vi "AG33XXX.constructor.vi"(0 "name":string, 2 "data in":string, 5 "error in (no error)":errorcluster) -> (14 "i ref out":refnum<vi>, 16 "data out":string, 19 "error out":errorcluster)   [LabVIEW 2014, in "AG33XXX.lvlib"]
doc: "Constructor of the AG33XXX class.\n\nLicense Agreement for this software:\n\nCopyright (C)\nGesellschaft für Schwerionenforschung, GSI\nPlanckstr. 1\n64291 Darmstadt\nGermany\n\nContact: D.Beck@gsi.de \n\nThis program is free software; you can redistribute it and/or modify it under the terms of the \nGNU General Public License as published by the Free Software Foundation; either version 2 of \nthe license, or (at your option) any later version.\n\nThis program is distributed in the hope that it will be useful, but WITHOUT ANY WARRANTY; \nwithout even the implied warranty of MERCHANTABILITY or FITNESS FOR A PARTICULAR PURPOSE. See the GNU General License for more details (http://www.gnu.org).\n\nGesellschaft für Schwerionenforschung, GSI\nPlanckstr. 1, 64291 Darmstadt, Germany\nFor all questions and ideas contact: M.Richter@gsi.de, H.Brand@gsi.de or D.Beck@gsi.de.\nLast update: 16-JUN-2004"
uses:
  AG33XXX.lvlib
  CS_Core/CSApplicationBaseClasses/DeviceBase/DeviceBase.myEventNames.ctl
  CS_Core/CSApplicationBaseClasses/AFGBase/AFGBase.myEventNames.ctl
  CS_Core/CSSystem/CSSystemLib/CSSystemLib.lvlib
  CS_Core/CSApplicationBaseClasses/AFGBase/AFGBase.lvlib
  CS_Core/CSApplicationBaseClasses/DeviceBase/DeviceBase.lvlib
  CS_Core/BaseProcess/BaseProcess.lvlib
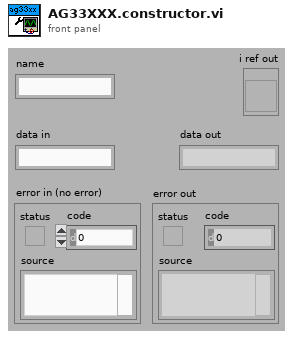
[diagram p1: front panel]
types:
  T1 = enum16{"SetAttribute", "GetAttribute", "CreateAttribute", "DestroyAttribute", "DestroyAllAtributes"}
  T2 = typedef "AFGBase.lvlib/AFGBase.myEventNames.ctl" = enum16{"lvmsg://SetFrequency", "lvmsg://GetFrequency", "lvmsg://SetAmplitude", "lvmsg://GetAmplitude", "lvmsg://SetPhase", "lvmsg://GetPhase", "lvmsg://SetDCOffset", "lvmsg://GetDCOffset", "lvmsg://SetWaveformType", "lvmsg://GetWaveformType", "lvmsg://SetOutputEnabled", "lvmsg://GetOutputEnabled", "lvmsg://SetWaveform", "lvmsg://GetWaveform", "lvmsg://SetTrigger", "lvmsg://GetTrigger", "lvmsg://SetWaveformParams", "lvmsg://GetWaveformParams"}
  T3 = typedef "DeviceBase.lvlib/DeviceBase.myEventNames.ctl" = enum16{"lvmsg://Initialize", "lvmsg://Close", "lvmsg://Configure", "lvmsg://Reset", "lvmsg://IDQuery"}
  T4 = typedef "BaseProcess.lvlib/BaseProcess.i attribute.ctl" = cluster{"EventStatus":string, "EventError":i32, "PresetEvtWatchD":i32, "PresetPdcWatchD":i32, "EventTimeout":i32, "PeriodicInterval":i32, "Interface":string[], "Address":string[], "Special":string[], "PeriodicError":i32, "PeriodicStatus":string, "SuperProc":string, "Descriptors":T5[], "CaseRef":refnum<vi>, "PdcRef":refnum<vi>, "Thread Ref":refnum<vi>, "eventErrorID":i32, "eventStatusID":i32, "periodicErrorID":i32, "periodicStatusID":i32, "pdcCtrID":i32}
  T5 = typedef "BaseProcess.lvlib/BaseProcess.descriptor definition.ctl" = cluster{"selector":string, "descriptor":T6}
  T6 = typedef "BaseProcess.lvlib/BaseProcess.descriptor string definition.ctl" = string
  T7 = typedef "AG33XXX.lvlib/AG33XXX.i attribute.ctl" = cluster{"Gauss_Offset":dbl}
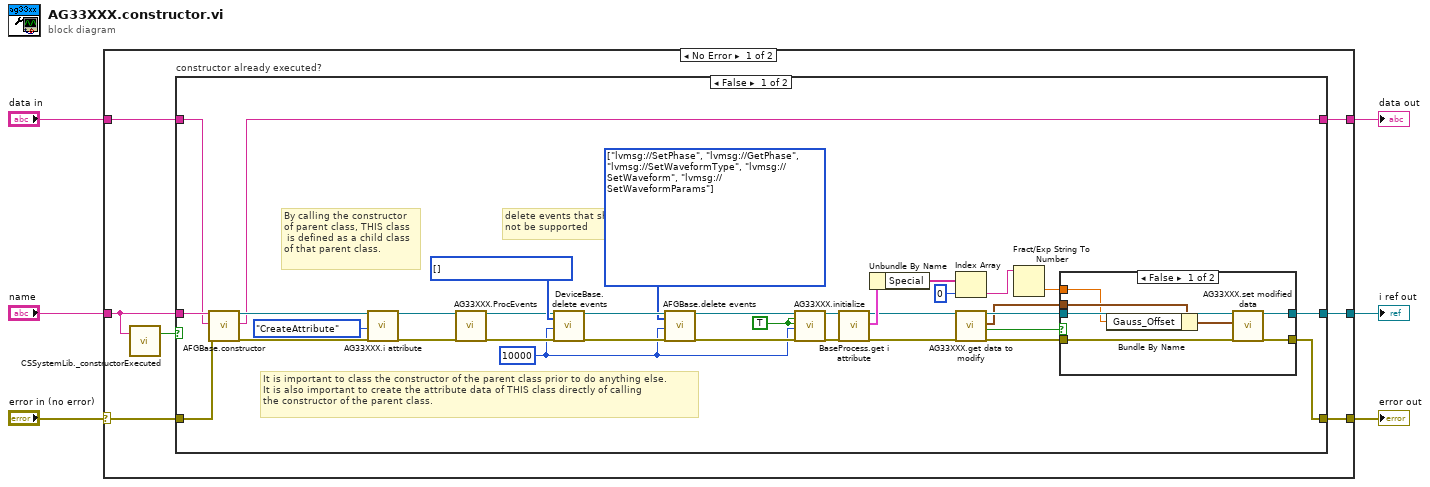
[diagram p0: block diagram]
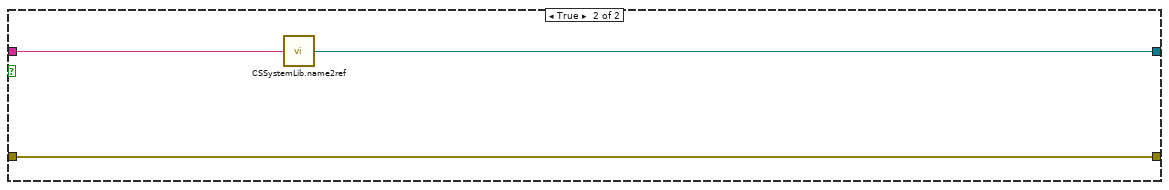
[diagram p3: hidden frame]
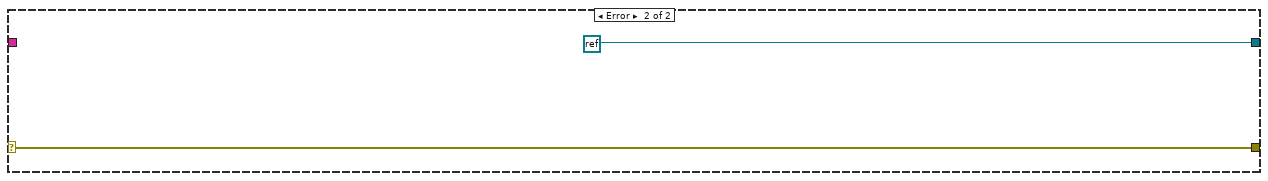
[diagram p4: hidden frame]
diagram:
  n1 = case shown="No Error" "error in (no error)" {
    selector: "error in (no error)" -> [w11 w60]
    tunnel: "name" -> [w10 _]
    tunnel: [w13 refnum<k0> refnum] -> w5
    tunnel: [w12 w60] -> w4
    tunnel: "data in" -> [w8 _]
    tunnel: [w7 _] -> w1
    frame No Error {
      n2 = call "CSSystemLib._constructorExecuted.vi"("name"=w10) -> ("constructor executed?"=w9:bool)  [unwired: 18 in]
      n3 = case "constructor already executed?" shown="False" w9 {
        tunnel: w10 -> [w44 w59]
        tunnel: [w21 w58] -> w13
        tunnel: [w20 w57] -> w12
        tunnel: w11 -> [w41 w57]
        tunnel: w8 -> [w40 _]
        tunnel: [w29 _] -> w7
        frame False {
          w34 = T2[] [enum."lvmsg://SetPhase", enum."lvmsg://GetPhase", enum."lvmsg://SetWaveformType", enum."lvmsg://SetWaveform", enum."lvmsg://SetWaveformParams"] items=["lvmsg://SetFrequency", "lvmsg://GetFrequency", "lvmsg://SetAmplitude", "lvmsg://GetAmplitude", "lvmsg://SetPhase", "lvmsg://GetPhase", "lvmsg://SetDCOffset", "lvmsg://GetDCOffset", "lvmsg://SetWaveformType", "lvmsg://GetWaveformType", "lvmsg://SetOutputEnabled", "lvmsg://GetOutputEnabled", "lvmsg://SetWaveform", "lvmsg://GetWaveform", "lvmsg://SetTrigger", "lvmsg://GetTrigger", "lvmsg://SetWaveformParams", "lvmsg://GetWaveformParams"] ("events")
          w39 = T3[] [] items=["lvmsg://Initialize", "lvmsg://Close", "lvmsg://Configure", "lvmsg://Reset", "lvmsg://IDQuery"] ("events")
          w31 = TRUE ("queryID")
          w30 = 10000 ("ms timeout (10000)")
          # "delete events that should\nnot be supported"
          # "It is important to class the constructor of the parent class prior to do anything else.\nIt is also important to create the attribute data of THIS class directly of calling\nthe constructor of the parent class."
          # "By calling the constructor\nof parent class, THIS class\n is defined as a child class\nof that parent class."
          n4 = call "AFGBase.constructor.vi"("name"=w44, "data in"=w40, "error in (no error)"=w41) -> ("i ref out"=w47:refnum<vi>, "data out"=w29:string, "error out"=w46:errorcluster)  [unwired: 14 in]
          n5 = call "AG33XXX.i attribute.vi"("VI Refnum"=w47, "Action"=T1."CreateAttribute", "error in (no error)"=w46) -> ("VI Refnum out"=w43:refnum<vi>, "error out"=w42:errorcluster)  [unwired: 14 in, 1 out]
          n6 = call "AG33XXX.ProcEvents.vi"("i ref in"=w43, "error in (no error)"=w42) -> ("i ref out"=w38:refnum<vi>, "error out"=w37:errorcluster)  [unwired: 16 in]
          n7 = call "DeviceBase.delete events.vi"("i ref in"=w38, "events"=w39, "ms timeout (10000)"=w30, "error in (no error)"=w37) -> ("i ref out"=w36:refnum<vi>, "error out"=w35:errorcluster)  [unwired: 13 in, 1 out]
          n8 = call "AFGBase.delete events.vi"("i ref in"=w36, "events"=w34, "ms timeout (10000)"=w30, "error in (no error)"=w35) -> ("i ref out"=w33:refnum<vi>, "error out"=w32:errorcluster)  [unwired: 13 in, 1 out]
          n9 = call "AG33XXX.initialize.vi"("i ref in"=w33, "queryID"=w31, "resetDevice"=w31, "ms timeout (10000)"=w30, "error in (no error)"=w32) -> ("i ref out"=w28:refnum<vi>, "error out"=w27:errorcluster)  [unwired: 11 in, 2 out]
          n10 = call "BaseProcess.get i attribute.vi"("i ref in"=w28, "error in (no error)"=w27) -> ("i ref out"=w23:refnum<vi>, "i attribute"=w26:T4, "error out"=w18:errorcluster)  [unwired: 15 in]
          n11 = Unbundle By Name(w26) -> ("Special"=w25:string[])
          n12 = Index Array(array=w25, index=0) -> (element=w15:string)
          n13 = call "AG33XXX.get data to modify.vi"("i ref in"=w23, "error in (no error)"=w18) -> ("i ref out"=w22:refnum<vi>, "i attribute"=w16:T7, "timed out"=w17:bool, "error out"=w19:errorcluster)  [unwired: 14 in]
          n14 = Fract/Exp String To Number(string=w15) -> (number=w14:dbl)  [unwired: 3 in, 1 out]
          n15 = case shown="False" w17 {
            tunnel: w22 -> [w54 w56]
            tunnel: [w53 w56] -> w21
            tunnel: [w52 w55] -> w20
            tunnel: w19 -> [w51 w55]
            tunnel: w16 -> [w50 _]
            tunnel: w14 -> [w48 _]
            frame False {
              n16 = Bundle By Name(cluster=w50, "Gauss_Offset"=w48) -> (w49:T7)
              n17 = call "AG33XXX.set modified data.vi"("i ref in"=w54, "i attribute"=w49, "error in (no error)"=w51) -> ("i ref out"=w53:refnum<vi>, "error out"=w52:errorcluster)  [unwired: 15 in]
            }
            frame True {
            }
          }
        }
        frame True {
          n18 = call "CSSystemLib.name2ref.vi"("name"=w59) -> ("obj refnum"=w58:refnum<vi>)
        }
      }
    }
    frame Error {
    }
  }
  "i ref out" <- w5
  "error out" <- w4
  "data out" <- w1
